vi "Draw-Circle.vi"() -> ()   [LabVIEW 2014]
panel:
  out "XY Graph":cluster{dbl[], dbl[]}(graph)
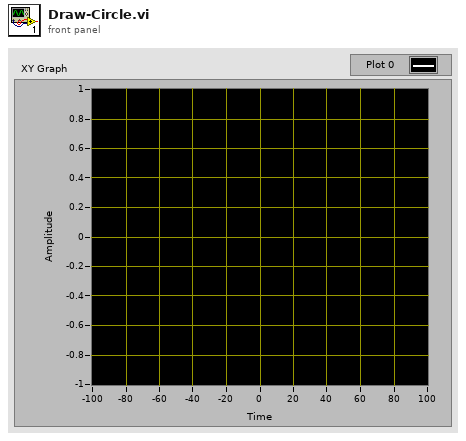
[diagram p1: front panel]
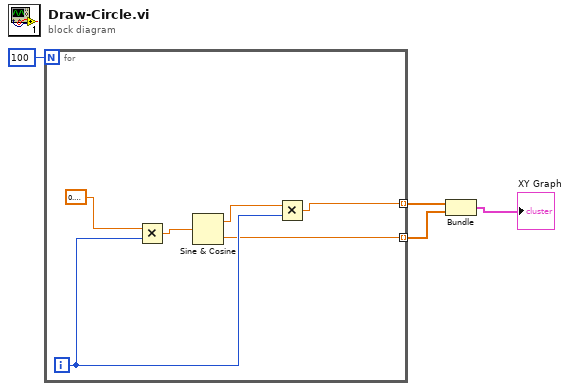
[diagram p0: block diagram]
diagram:
  n1 = for {
    N: 100 -> [_]
    tunnel: [w6] -> w3 mode=indexing
    tunnel: [w5] -> w2 mode=indexing
    i -> [w7]
    n2 = Multiply(x=0.3183098861837907, y=w7) -> (x*y=w9:dbl)
    n3 = Sine & Cosine(0:w9) -> (1:w8:dbl, 2:w5:dbl)
    n4 = Multiply(x=w8, y=w7) -> (x*y=w6:dbl)
  }
  n5 = Bundle(w3, w2) -> (→"XY Graph":cluster{dbl[], dbl[]})  [unwired: 1 in]
